vi "Read T Controller Settings.vi"(8 "error in (no error)":errorcluster, 11 "Temperature controller in":refnum<class "Temperature controller.lvclass">) -> (0 "error out":errorcluster, 1 "Heater level":dbl, 2 "Heater mode":T1(ring), 3 "Temperature controller out":refnum<class "Temperature controller.lvclass">, 4 "PID":cluster{"P":dbl, "I":dbl, "D":dbl}, 5 "Hater range":dbl, 7 "Set point":dbl)   [LabVIEW 2015, in "Temperature controller.lvclass"]
uses:
  Temperature controller.lvclass
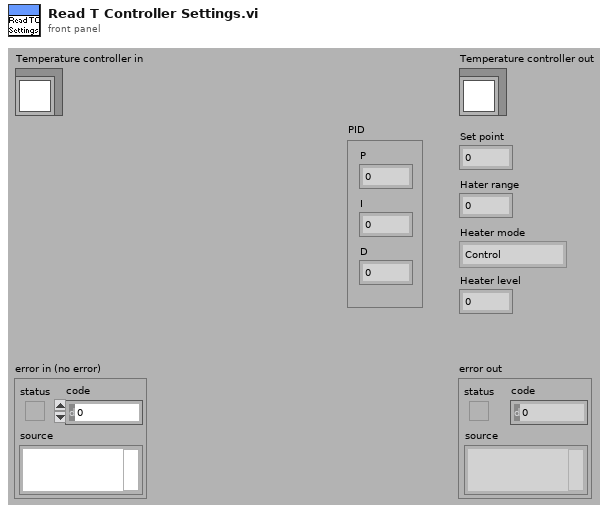
[diagram p1: front panel]
types:
  T1 = enum16{"Control", "Monitor", "Manual Heat", "Controller is in OFF mode", "Autotune is in progress"}
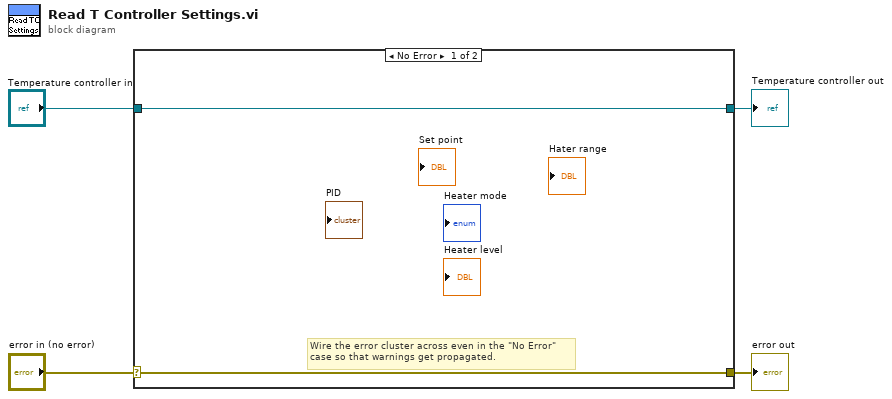
[diagram p0: block diagram]
diagram:
  n1 = case shown="No Error" "error in (no error)" {
    selector: "error in (no error)" -> [w5 w8]
    tunnel: [w5 w8] -> w3
    tunnel: [w6 w7] -> w1
    tunnel: "Temperature controller in" -> [w6 w7]
    frame No Error {
      # "Wire the error cluster across even in the \"No Error\"\ncase so that warnings get propagated."
    }
    frame Error {
    }
  }
  "error out" <- w3
  "Temperature controller out" <- w1
